vi "Pelletron_Queue.vi"(11 "AccelNET.lvlib:PelletronStatus.lvclass":refnum<class "PelletronStatus.lvclass">) -> ()   [LabVIEW 2012, in "AccelNET.lvlib" / "PelletronStatus.lvclass"]
uses:
  PelletronStatus.lvclass
  PelletronStatus.lvclass/PelletronStatus.ctl
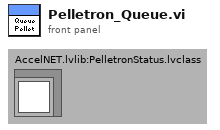
[diagram p1: front panel]
types:
  T1 = typedef "Interface.lvlib/Pelletron.ctl" = cluster{"Timestamp":u64, "High Voltage":sgl, "Vacuum Pressure":sgl, "Column Current":sgl, "Chain Current":sgl, "- High Voltage Supply":dbl, "+ High Voltage Supply":dbl, "Radiation":dbl, "Lost Charge":dbl, "Control High Voltage":dbl, "HV Control Difference":dbl}
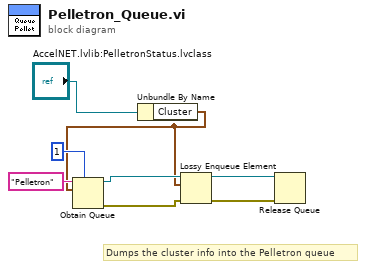
[diagram p0: block diagram]
diagram:
  # "Dumps the cluster info into the Pelletron queue"
  n1 = Unbundle By Name("AccelNET.lvlib:PelletronStatus.lvclass") -> ("Cluster"=w4:T1)
  n2 = Obtain Queue(max queue size (-1, unlimited)=1, name (unnamed)="Pelletron", element data type=w4) -> (queue out=w5:refnum<queue>, error out=w3:errorcluster)  [unwired: 2 in, 1 out]
  n3 = Lossy Enqueue Element(queue=w5, element=w4, error in (no error)=w3) -> (queue out=w1:refnum<queue>, error out=w2:errorcluster)  [unwired: 2 out]
  n4 = Release Queue(queue=w1, error in (no error)=w2) -> ()  [unwired: 1 in, 3 out]
